vi "TCP-Send Command Receive String (CRLF).vi"(0 "PXI Address":string, 5 "Port":i32, 7 "Command":string, 9 "timeout (ms)":i32=5000, 11 "error in (no error)":errorcluster) -> (4 "data":string, 10 "result":i32, 15 "error out":errorcluster)   [LabVIEW 2020]
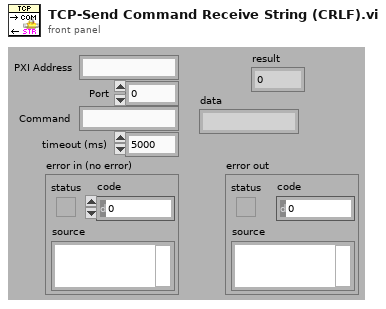
[diagram p1: front panel]
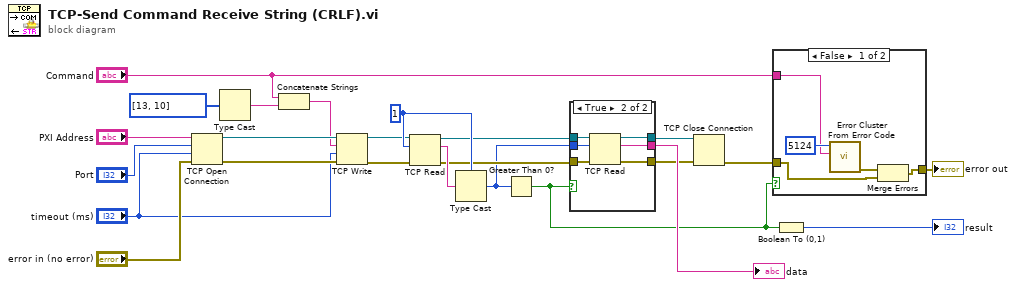
[diagram p0: block diagram]
diagram:
  w15 = u8 1
  n1 = TCP Open Connection(address="PXI Address", remote port or service name="Port", timeout ms (60000)="timeout (ms)", error in (no error)="error in (no error)") -> (connection ID=w20:refnum<k5>, error out=w21:errorcluster)  [unwired: 1 in]
  n2 = Type Cast(x=u8[] [13, 10]) -> (*(type *) &x=w5:string)  [unwired: 1 in]
  n3 = Concatenate Strings("Command", w5) -> (w3:string)
  n4 = TCP Write(connection ID=w20, data in=w3, error in (no error)=w21, 9:"timeout (ms)") -> (connection ID out=w14:refnum<k5>, error out=w13:errorcluster)  [unwired: 1 out]
  n5 = TCP Read(connection ID=w14, bytes to read=w15, error in (no error)=w13) -> (connection ID out=w11:refnum<k5>, data out=w16:string, error out=w12:errorcluster)  [unwired: 2 in]
  n6 = Type Cast(type=w15, x=w16) -> (*(type *) &x=w8:u8)
  n7 = Greater Than 0?(x=w8) -> (x > 0?=w1:bool)
  n8 = case shown="True" w1 {
    tunnel: [_ w32] -> w9
    tunnel: [w26 w31] -> w7
    tunnel: w11 -> [w25 w30]
    tunnel: w12 -> [w26 w29]
    tunnel: w8 -> [_ w28]
    tunnel: [w25 w27] -> w10
    frame False {
    }
    frame True {
      n9 = TCP Read(connection ID=w30, bytes to read=w28, error in (no error)=w29) -> (connection ID out=w27:refnum<k5>, data out=w32:string, error out=w31:errorcluster)  [unwired: 2 in]
    }
  }
  "data" <- w9
  n10 = TCP Close Connection(connection ID=w10, error in (no error)=w7) -> (error out=w17:errorcluster)  [unwired: 1 in, 1 out]
  n11 = case shown="False" w1 {
    tunnel: [w34 w38] -> w18
    tunnel: w17 -> [w33 w38]
    tunnel: "Command" -> [w35 _]
    frame False {
      n12 = call <vilib>:"Error Cluster From Error Code.vi"("error message (\"\")"=w35, "error code (0)"=5124) -> ("error out"=w37:errorcluster)  [unwired: 7 in]
      n13 = Merge Errors(w37, w33) -> (w34:errorcluster)
    }
    frame True {
    }
  }
  "error out" <- w18
  n14 = Boolean To (0,1)(Boolean=w1) -> (0, 1=→"result":i16)
